vi "Disable Heating.vi"(8 "error in (no error)":errorcluster, 10 "Start Time":timestamp, 11 "Thermal Chamber Response Simlator In":refnum<class "Thermal Chamber Response Simlator.lvclass">) -> (0 "error out":errorcluster, 3 "Thermal Chamber Response Simlator Out":refnum<class "Thermal Chamber Response Simlator.lvclass">)   [LabVIEW 2020, in "Thermal Chamber Response Simlator.lvclass"]
uses:
  Thermal Chamber Response Simlator.lvclass
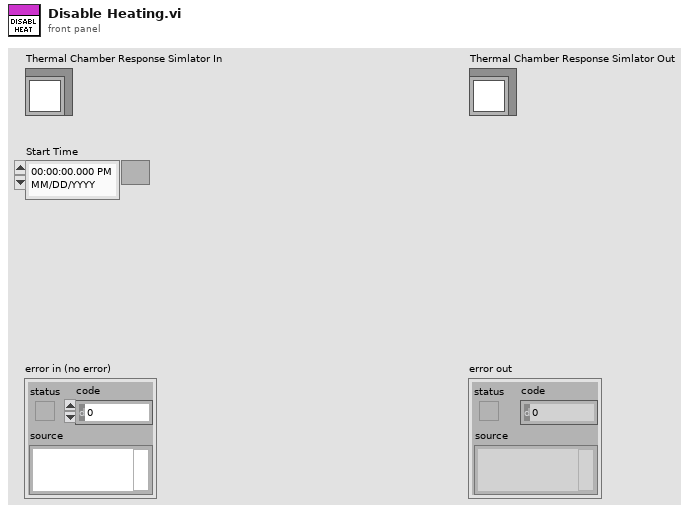
[diagram p1: front panel]
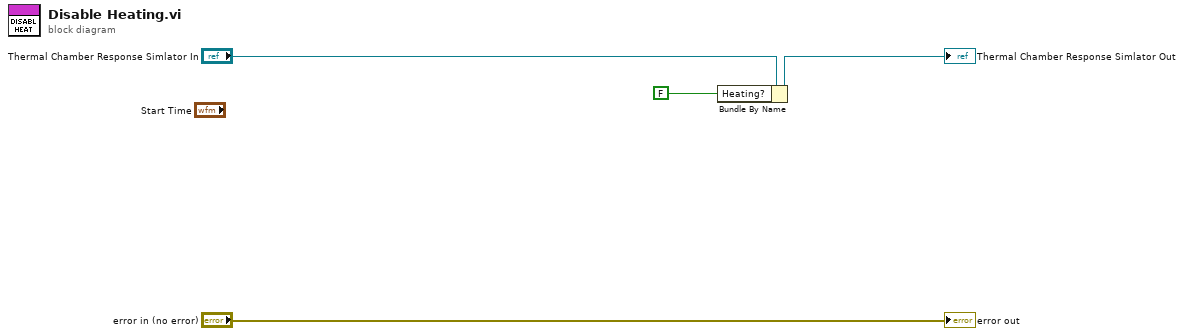
[diagram p0: block diagram]
diagram:
  n1 = Bundle By Name(cluster="Thermal Chamber Response Simlator In", "Heating?"=FALSE) -> (→"Thermal Chamber Response Simlator Out":refnum<class "Thermal Chamber Response Simlator.lvclass">)
  "error out" <- "error in (no error)"
